vi "Variant_SetName.vi"(10 "Name":string, 11 "Variant":variant) -> (3 "Named Variant":variant)   [LabVIEW 2017, in "JSONtext.lvlib"]
uses:
  JSONtext.lvlib
  <vilib>/LabVIEW Open Source Project/Data Manipulation/TypeDescriptor/OpenDescriptor.lvlib
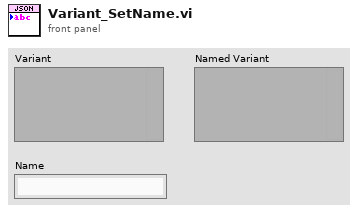
[diagram p1: front panel]
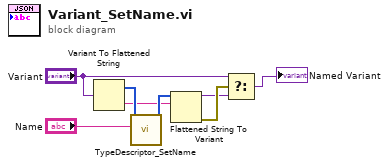
[diagram p0: block diagram]
diagram:
  n1 = Variant To Flattened String(Variant="Variant") -> (data string=w5:string, 1:w7:i16[])
  n2 = call <vilib>:"TypeDescriptor_SetName.vi"("name"="Name", "type descriptor"=w7) -> ("type descriptor dup"=w8:i16[])  [unwired: 7 in, 2 out]
  n3 = Flattened String To Variant(6:w5, 7:w8) -> (0:w3:errorcluster, 3:w2:variant)  [unwired: 1 in]
  n4 = Select(t="Variant", s=w3, f=w2) -> (s? t:f=→"Named Variant":variant)
